vi "Send Mouseover Panel Object.vi"(7 "Message Priority (Normal)":T2=enum."Normal", 8 "error in (no error)":errorcluster, 10 "Coords":T1, 11 "Message Enqueuer":refnum<class "Message Enqueuer.lvclass">) -> (0 "error out":errorcluster, 3 "Message Enqueuer out":refnum<class "Message Enqueuer.lvclass">)   [LabVIEW 2018, in "Pane Relief Main UI.lvlib" / "Mouseover Panel Object Msg.lvclass"]
doc: "This VI sends the message to an actor."
uses:
  <resource>/dialog/QuickDrop/plugins/PaneRelief/Classes/Pane Relief Main UI/Pane Relief Main UI Messages/Mouseover Panel Object Msg/Mouseover Panel Object Msg.lvclass
  <vilib>/ActorFramework/Message Enqueuer/Message Enqueuer.lvclass
  <vilib>/ActorFramework/Message Enqueuer/Message Priority.ctl
  <vilib>/Utility/miscctls.llb/LVPoint32TypeDef.ctl
  C:/Program Files (x86)/National Instruments/LabVIEW 2018/vi.lib/ActorFramework/Message/Message.lvclass
  <resource>/dialog/QuickDrop/plugins/PaneRelief/Classes/Pane Relief Main UI/Pane Relief Main UI Messages/Mouseover Panel Object Msg/Mouseover Panel Object Msg.lvclass/Mouseover Panel Object Msg.ctl
  <vilib>/ActorFramework/Message Enqueuer/Message Enqueuer.lvclass/Message Enqueuer.ctl
  <vilib>/ActorFramework/Message Priority Queue/Priority Enqueue.vi
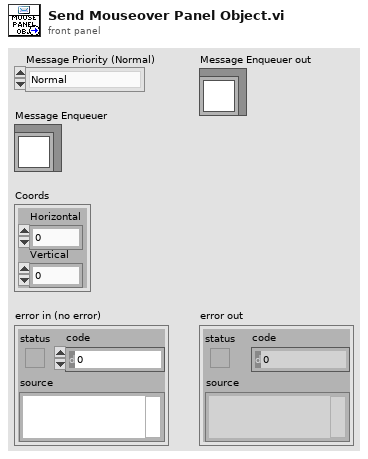
[diagram p1: front panel]
types:
  T1 = typedef "LVPoint32TypeDef.ctl" = cluster{"Horizontal":i32, "Vertical":i32}
  T2 = typedef "Actor Framework.lvlib/Message Enqueuer.lvclass/Message Priority.ctl" = enum16{"Low", "Normal", "High"}
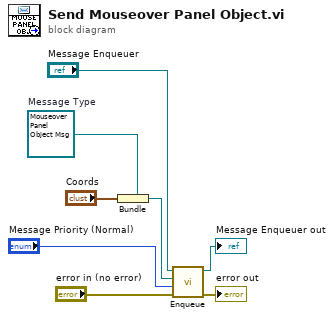
[diagram p0: block diagram]
diagram:
  w2 = refnum<class "Mouseover Panel Object Msg.lvclass"> refnum  # Message Type
  n1 = Bundle(cluster=w2, "Coords") -> (w3:refnum<class "Mouseover Panel Object Msg.lvclass">)
  n2 = call <vilib>:"Enqueue.vi"("error in (no error)"="error in (no error)", "Message Priority (Normal)"="Message Priority (Normal)", "Message"=w3, "Message Enqueuer in"="Message Enqueuer") -> ("error out"=→"error out":errorcluster, "Message Enqueuer out"=→"Message Enqueuer out":refnum<class "Message Enqueuer.lvclass">)  [unwired: 6 in]
